vi "根据参考点计算一组标准坐标.vi"(4 "Y方向间隔(mm)":dbl, 6 "X方向间隔(mm)":dbl, 7 "行数":i32=4, 9 "Point (Pixels)":cluster{"X":sgl, "Y":sgl}, 10 "列数":i32=6) -> (3 "所有点投影 2":cluster{"Distance":dbl, "Distance":dbl}[](array[cluster]))   [LabVIEW 2014]
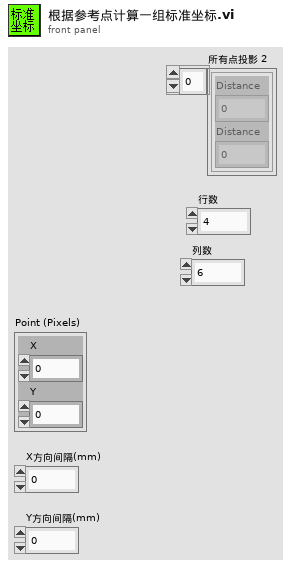
[diagram p1: front panel]
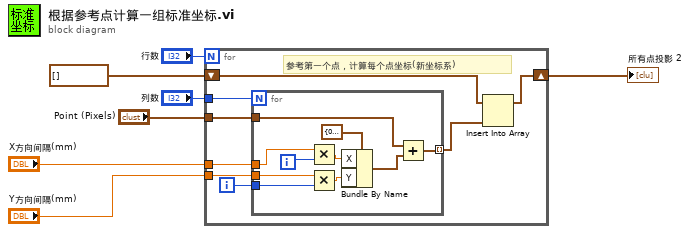
[diagram p0: block diagram]
diagram:
  n1 = for {
    N: "行数" -> [_]
    tunnel: "Point (Pixels)" -> [w14]
    tunnel: "X方向间隔(mm)" -> [w13]
    tunnel: "Y方向间隔(mm)" -> [w15]
    shift-right: [w11] -> w5
    shift-left: cluster{"Distance":dbl, "Distance":dbl}[] [] ("所有点投影 3") -> [w12]
    tunnel: "列数" -> [w8]
    i -> [w10]
    # "参考第一个点，计算每个点坐标(新坐标系)"
    n2 = for {
      N: w8 -> [_]
      tunnel: w15 -> [w25]
      tunnel: w14 -> [w24]
      tunnel: w13 -> [w20]
      tunnel: w10 -> [w21]
      tunnel: [w17] -> w9 mode=indexing
      i -> [w19]
      n3 = Multiply(x=w20, y=w19) -> (x*y=w18:dbl)
      n4 = Multiply(x=w25, y=w21) -> (x*y=w22:dbl)
      n5 = Bundle By Name(cluster=cluster{"X":sgl, "Y":sgl} {"X"=0.0, "Y"=0.0} ("Point1 (Pixels)"), "X"=w18, "Y"=w22) -> (w23:cluster{"X":sgl, "Y":sgl})
      n6 = Add(x=w24, y=w23) -> (x+y=w17:cluster{"X":sgl, "Y":sgl})
    }
    n7 = Insert Into Array(array=w12, new element=w9) -> (w11:cluster{"Distance":dbl, "Distance":dbl}[])  [unwired: 1 in]
  }
  "所有点投影 2" <- w5
